vi "Get Sweep.vi"(0 "Sweep Name":string, 11 "error in (no error)":errorcluster) -> (4 "Grid":T1, 6 "Sweep not found?":bool, 15 "error out":errorcluster)   [LabVIEW 2023, in "RFFixtureCharact.RFPM.lvlib" / "Vector 18GHz Path.lvclass"]
uses:
  Vector 18GHz Path.lvclass
  Path Groups/Vector Path Group/Type Definitions/Sweep.ctl
  Vector 18GHz Path.lvclass/Vector 18GHz Path.ctl
  Common/RFCalAndFixtureCharact.Common.lvlib
  Path Groups/Vector Path Group/Vector 18GHz Path Group.lvclass
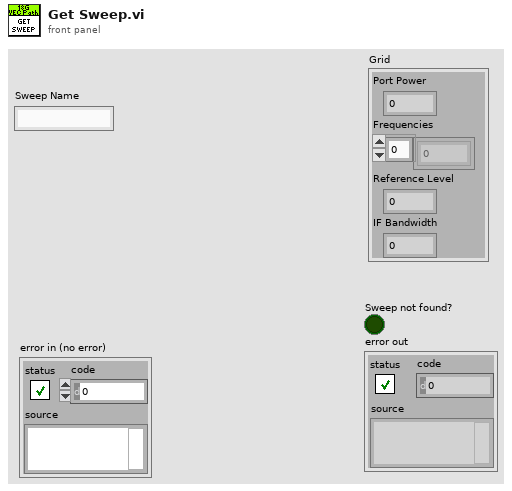
[diagram p1: front panel]
types:
  T1 = typedef "RFFixtureCharact.RFPM.lvlib/Vector 18GHz Path Group.lvclass/Sweep.ctl" = cluster{"Port Power":dbl, "Frequencies":dbl[], "Reference Level":dbl, "IF Bandwidth":dbl}
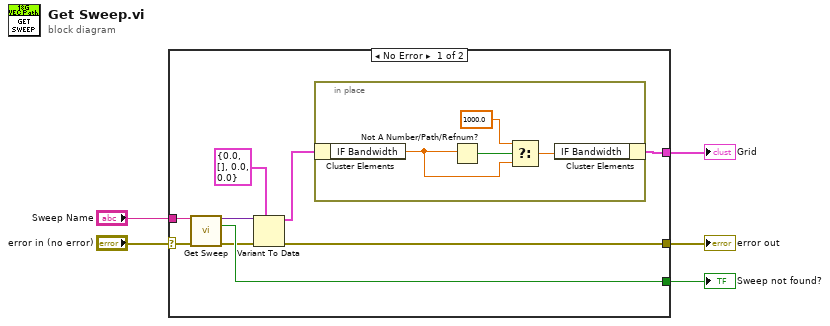
[diagram p0: block diagram]
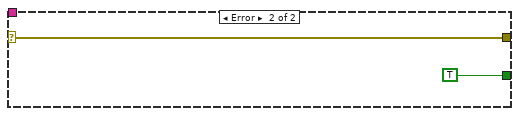
[diagram p2: hidden frame]
diagram:
  n1 = case shown="No Error" "error in (no error)" {
    selector: "error in (no error)" -> [w10 w19]
    tunnel: "Sweep Name" -> [w14 _]
    tunnel: [w8 w19] -> w4
    tunnel: [w13 TRUE ("Sweep not found?")] -> w3
    tunnel: [w6 _] -> w2
    frame No Error {
      n2 = call "Get Sweep.vi"("Sweep Name"=w14, "error in (no error)"=w10) -> ("Variant"=w11:variant, "Sweep not found?"=w13:bool, "error out"=w9:errorcluster)  [unwired: 11 in]
      n3 = Variant To Data(error in=w9, type=T1 {"Port Power"=0.0, "Frequencies"=[], "Reference Level"=0.0, "IF Bandwidth"=0.0} ("Grid"), Variant=w11) -> (data=w7:T1, error out=w8:errorcluster)
      n4 = in-place {
        n5 = in-place-cluster #1(w7) -> ("IF Bandwidth"=w16:dbl)
        n6 = Not A Number/Path/Refnum?(number/path/refnum=w16) -> (NaN/Path/Refnum?=w15:bool)
        n7 = Select(t=1000.0, s=w15, f=w16) -> (s? t:f=w17:dbl)
        n8 = in-place-cluster #1("IF Bandwidth"=w17) -> (w6:T1)
      }
    }
    frame Error {
    }
  }
  "error out" <- w4
  "Sweep not found?" <- w3
  "Grid" <- w2
